vi "Buffer Setpoints.vi"(8 "error in (no error)":errorcluster, 11 "Model in":refnum<class "Model.lvclass">) -> (0 "error out":errorcluster, 3 "Model out":refnum<class "Model.lvclass">)   [LabVIEW 2016]
uses:
  Model.lvclass
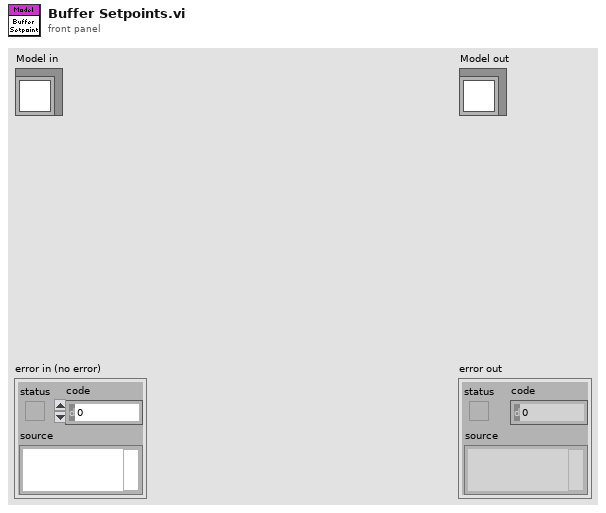
[diagram p1: front panel]
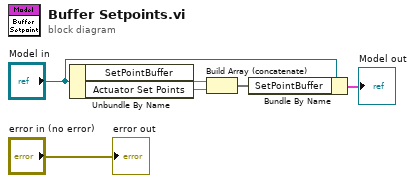
[diagram p0: block diagram]
diagram:
  n1 = Unbundle By Name("Model in") -> ("SetPointBuffer"=w6, "Actuator Set Points"=w5)
  n2 = Build Array (concatenate)(w6, w5) -> (w3:void[])
  n3 = Bundle By Name(cluster="Model in", "SetPointBuffer"=w3) -> (→"Model out":cluster{})
  "error out" <- "error in (no error)"
